vi "QueryCustomDevices.vi"(8 "error in (no error)":errorcluster, 11 "Target Reference In":refnum<k24>) -> (0 "error out":errorcluster, 2 "Custom Devices":string[](array[string]), 3 "Target Reference out":refnum<k24>)   [LabVIEW 2017, in "VeriStandTestUtilities.lvlib"]
uses:
  VeriStandTestUtilities.lvlib
  NationalInstruments.VeriStand.SystemDefinitionAPI
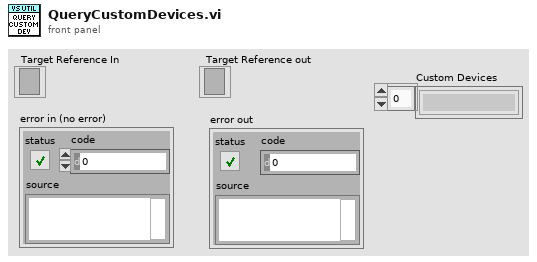
[diagram p1: front panel]
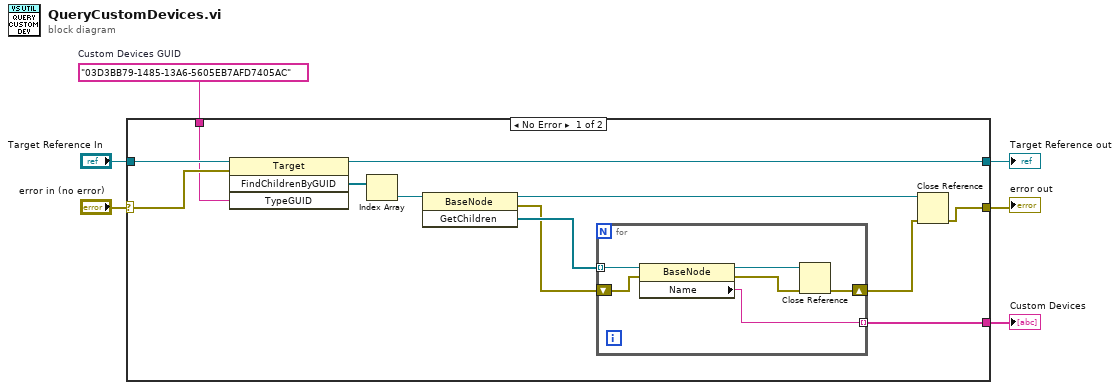
[diagram p0: block diagram]
diagram:
  w2 = "03D3BB79-1485-13A6-5605EB7AFD7405AC"  # Custom Devices GUID
  n1 = case shown="No Error" "error in (no error)" {
    selector: "error in (no error)" -> [w17 w26]
    tunnel: [w8 w26] -> w5
    tunnel: "Target Reference In" -> [w18 w25]
    tunnel: [w14 w25] -> w3
    tunnel: w2 -> [w16 _]
    tunnel: [w7 _] -> w1
    frame No Error {
      n2 = invoke class="Target" method="FindChildrenByGUID"(reference=w18, error in=w17, "TypeGUID"=w16) -> (reference out=w14:refnum<k24>, "FindChildrenByGUID"=w15:refnum<k24>[])  [unwired: 1 in, 2 out]
      n3 = Index Array(array=w15) -> (element=w13:refnum<k24>)  [unwired: 1 in]
      n4 = invoke class="BaseNode" method="GetChildren"(reference=w13) -> (reference out=w12:refnum<k24>, error out=w10:errorcluster, "GetChildren"=w11:refnum<k24>[])  [unwired: 2 in]
      n5 = for {
        tunnel: w11 -> [w24] mode=indexing
        shift-right: [w23] -> w9
        shift-left: w10 -> [w21]
        tunnel: [w19] -> w7 mode=indexing
        n6 = property class="BaseNode"(reference=w24, error in=w21) -> (reference out=w22:refnum<k24>, error out=w20:errorcluster, "Name"=w19:string)
        n7 = Close Reference(reference=w22, error in (no error)=w20) -> (error out=w23:errorcluster)
      }
      n8 = Close Reference(reference=w12, error in (no error)=w9) -> (error out=w8:errorcluster)
    }
    frame Error {
    }
  }
  "Target Reference out" <- w3
  "error out" <- w5
  "Custom Devices" <- w1
